vi "Record data into spreadsheet.vi"(1 "Error In":errorcluster, 2 "Append?":bool, 3 "Data":dbl[][](array[numeric]) format="%0.2f") -> (0 "Error Out":errorcluster)   [LabVIEW 2015]
uses:
  <vilib>/Utility/file.llb/Write Delimited Spreadsheet (DBL).vi
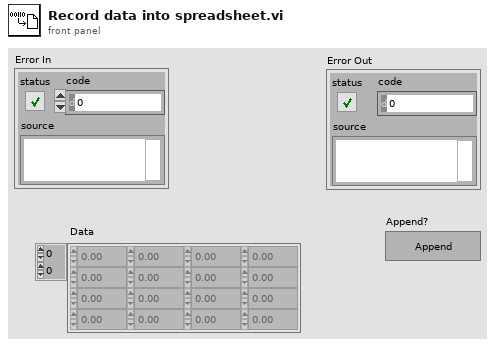
[diagram p1: front panel]
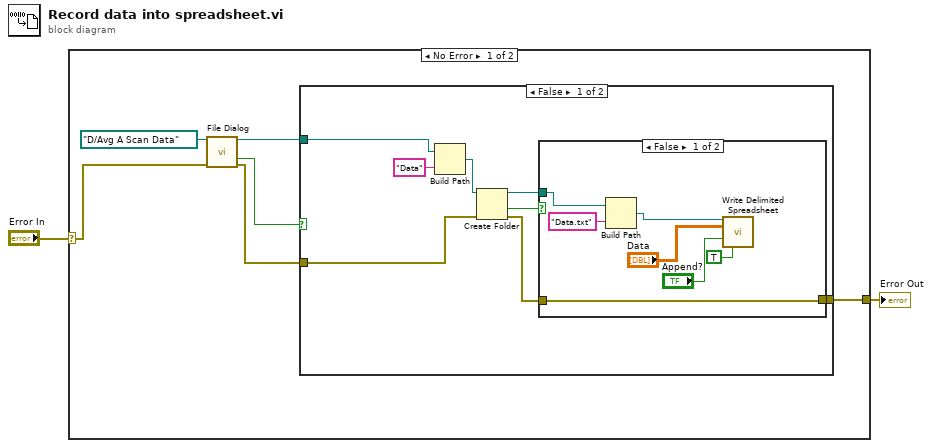
[diagram p0: block diagram]
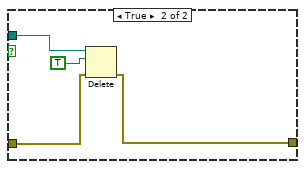
[diagram p2: hidden frame]
diagram:
  n1 = case shown="No Error" "Error In" {
    selector: "Error In" -> [w5 w29]
    tunnel: [w3 w29] -> w1
    frame No Error {
      n2 = call "File Dialog"("start path"=path "D:/Avg A Scan Data", "error in"=w5) -> ("selected path"=w7:path, "cancelled"=w8:bool, "error out"=w4:errorcluster)  [unwired: 10 in, 1 out]
      n3 = case shown="False" w8 {
        tunnel: w7 -> [w16 _]
        tunnel: w4 -> [w9 w28]
        tunnel: [w12 w28] -> w3
        frame False {
          n4 = Build Path(base path=w16, name or relative path="Data") -> (appended path=w15:path)
          n5 = Create Folder(path (use dialog)=w15, error in=w9) -> (created path=w13:path, cancelled=w14:bool, error out=w11:errorcluster)  [unwired: 1 in]
          n6 = case shown="False" w14 {
            tunnel: w13 -> [w21 w27]
            tunnel: w11 -> [w23 w25]
            tunnel: [w23 w24] -> w12
            frame False {
              n7 = Build Path(base path=w21, name or relative path="Data.txt") -> (appended path=w20:path)
              n8 = call-poly <vilib>:"Write Delimited Spreadsheet.vi"("file path (dialog if empty)"=w20, "2D data"="Data", "append to file? (F)"="Append?", "transpose? (F)"=TRUE ("transpose? (no:F)")) -> ()  [unwired: 10 in, 2 out]
            }
            frame True {
              n9 = Delete(path (use dialog)=w27, entire hierarchy (F)=TRUE ("confirm (F)"), error in=w25) -> (error out=w24:errorcluster)  [unwired: 2 in, 2 out]
            }
          }
        }
        frame True {
        }
      }
    }
    frame Error {
    }
  }
  "Error Out" <- w1
